vi "[GV]_IMU roll.vi"() -> ()   [LabVIEW 2016]
panel:
  in  "IMU roll":dbl
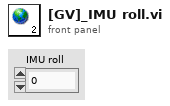
[diagram p1: front panel]
diagram:
